vi "Otsu分割算法.vi"() -> ()   [LabVIEW 2018]
uses:
  <vilib>/Utility/error.llb/DialogType.ctl
  <vilib>/vision/NI_Vision_Development_Module.lvlib
  Dll/Otsu.dll
panel:
  in  "保存":bool
  out "像素当量单位":string
  out "像素当量":string
  out "是否进行像素标定":bool
  in  "单帧回看":bool
  out "火焰帧数":string
  in  "重新选择":bool
  in  "火焰详细参数":bool
  out "叠加部分":string
  out "单帧部分":string
  out "原图":T1(plugin-control)
  in  "返回主界面":bool
  in  "程序停止":bool
  out "Progress Bar":i32(slide) max=241 scale=-1.0..241.0
  out "单帧火焰":T1(plugin-control)
  out "叠加火焰":T1(plugin-control)
  # "基于Otsu算法的炮口火焰分割"
  # "火\n焰\n参\n数"
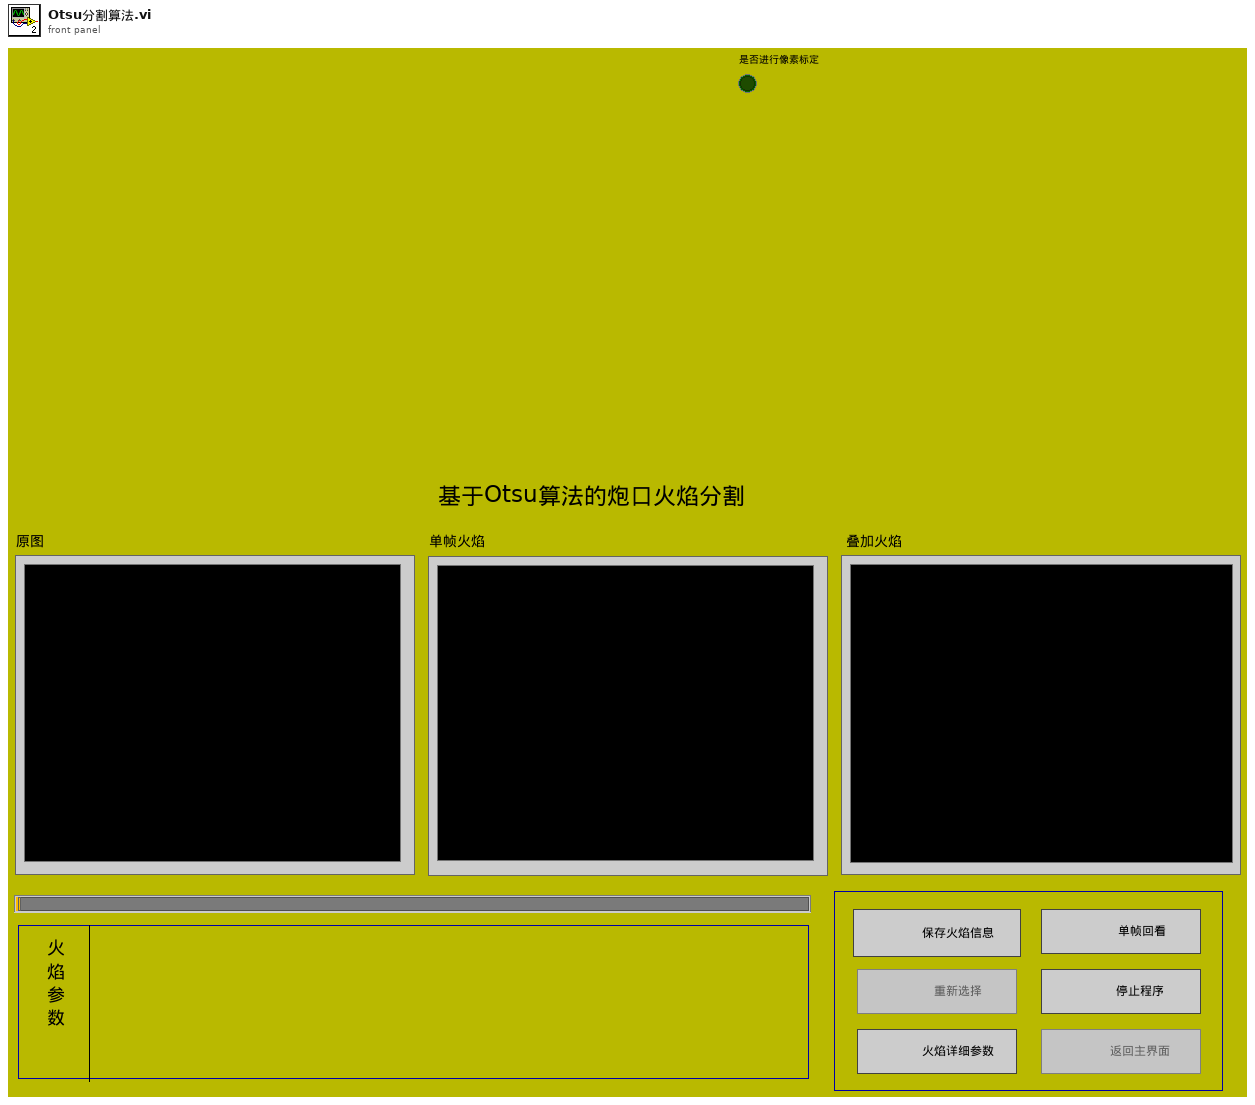
[diagram p1: front panel]
types:
  T1 = typedef "IMAQ Image.ctl" = refnum<image>
  T2 = enum8{"Enabled", "Disabled", "Disabled and Grayed Out"}
  T3 = enum32{"Invalid", "Standard", "Closed", "Hidden", "Minimized", "Maximized"}
  T4 = typedef "DialogType.ctl" = u16
  T5 = typedef "Image Type" = u32
  T6 = typedef "IMAQ AVI2 Refnum.ctl" = refnum<k20>
  T7 = cluster{"Width":u32, "Height":u32, "Frames Per Second":u32, "Codec":string, "Has Data":bool}
  T8 = typedef "ROI Descriptor" = cluster{"Global Rectangle":i32[], "Contours":cluster{"ID":enum32{"External", "Internal"}, "Type":u32, "Coordinates":i32[]}[]}
  T9 = cluster{"Area":dbl, "Number of Holes":dbl, "Bounding Rect":cluster{"Left":dbl, "Top":dbl, "Right":dbl, "Bottom":dbl}, "Center of Mass":cluster{"X":dbl, "Y":dbl}, "Orientation":dbl, "Dimensions":cluster{"Width":dbl, "Height":dbl}}[]
  T10 = cluster{"Particle Reports (Pixels)[0]":cluster{"Area":dbl, "Number of Holes":dbl, "Bounding Rect":cluster{"Left":dbl, "Top":dbl, "Right":dbl, "Bottom":dbl}, "Center of Mass":cluster{"X":dbl, "Y":dbl}, "Orientation":dbl, "Dimensions":cluster{"Width":dbl, "Height":dbl}}, "Particle Reports (Pixels)[1]":cluster{"Area":dbl, "Number of Holes":dbl, "Bounding Rect":cluster{"Left":dbl, "Top":dbl, "Right":dbl, "Bottom":dbl}, "Center of Mass":cluster{"X":dbl, "Y":dbl}, "Orientation":dbl, "Dimensions":cluster{"Width":dbl, "Height":dbl}}, "Particle Reports (Pixels)[2]":cluster{"Area":dbl, "Number of Holes":dbl, "Bounding Rect":cluster{"Left":dbl, "Top":dbl, "Right":dbl, "Bottom":dbl}, "Center of Mass":cluster{"X":dbl, "Y":dbl}, "Orientation":dbl, "Dimensions":cluster{"Width":dbl, "Height":dbl}}, "Particle Reports (Pixels)[3]":cluster{"Area":dbl, "Number of Holes":dbl, "Bounding Rect":cluster{"Left":dbl, "Top":dbl, "Right":dbl, "Bottom":dbl}, "Center of Mass":cluster{"X":dbl, "Y":dbl}, "Orientation":dbl, "Dimensions":cluster{"Width":dbl, "Height":dbl}}, "Particle Reports (Pixels)[4]":cluster{"Area":dbl, "Number of Holes":dbl, "Bounding Rect":cluster{"Left":dbl, "Top":dbl, "Right":dbl, "Bottom":dbl}, "Center of Mass":cluster{"X":dbl, "Y":dbl}, "Orientation":dbl, "Dimensions":cluster{"Width":dbl, "Height":dbl}}, "Particle Reports (Pixels)[5]":cluster{"Area":dbl, "Number of Holes":dbl, "Bounding Rect":cluster{"Left":dbl, "Top":dbl, "Right":dbl, "Bottom":dbl}, "Center of Mass":cluster{"X":dbl, "Y":dbl}, "Orientation":dbl, "Dimensions":cluster{"Width":dbl, "Height":dbl}}, "Particle Reports (Pixels)[6]":cluster{"Area":dbl, "Number of Holes":dbl, "Bounding Rect":cluster{"Left":dbl, "Top":dbl, "Right":dbl, "Bottom":dbl}, "Center of Mass":cluster{"X":dbl, "Y":dbl}, "Orientation":dbl, "Dimensions":cluster{"Width":dbl, "Height":dbl}}, "Particle Reports (Pixels)[7]":cluster{"Area":dbl, "Number of Holes":dbl, "Bounding Rect":cluster{"Left":dbl, "Top":dbl, "Right":dbl, "Bottom":dbl}, "Center of Mass":cluster{"X":dbl, "Y":dbl}, "Orientation":dbl, "Dimensions":cluster{"Width":dbl, "Height":dbl}}, "Particle Reports (Pixels)[8]":cluster{"Area":dbl, "Number of Holes":dbl, "Bounding Rect":cluster{"Left":dbl, "Top":dbl, "Right":dbl, "Bottom":dbl}, "Center of Mass":cluster{"X":dbl, "Y":dbl}, "Orientation":dbl, "Dimensions":cluster{"Width":dbl, "Height":dbl}}}
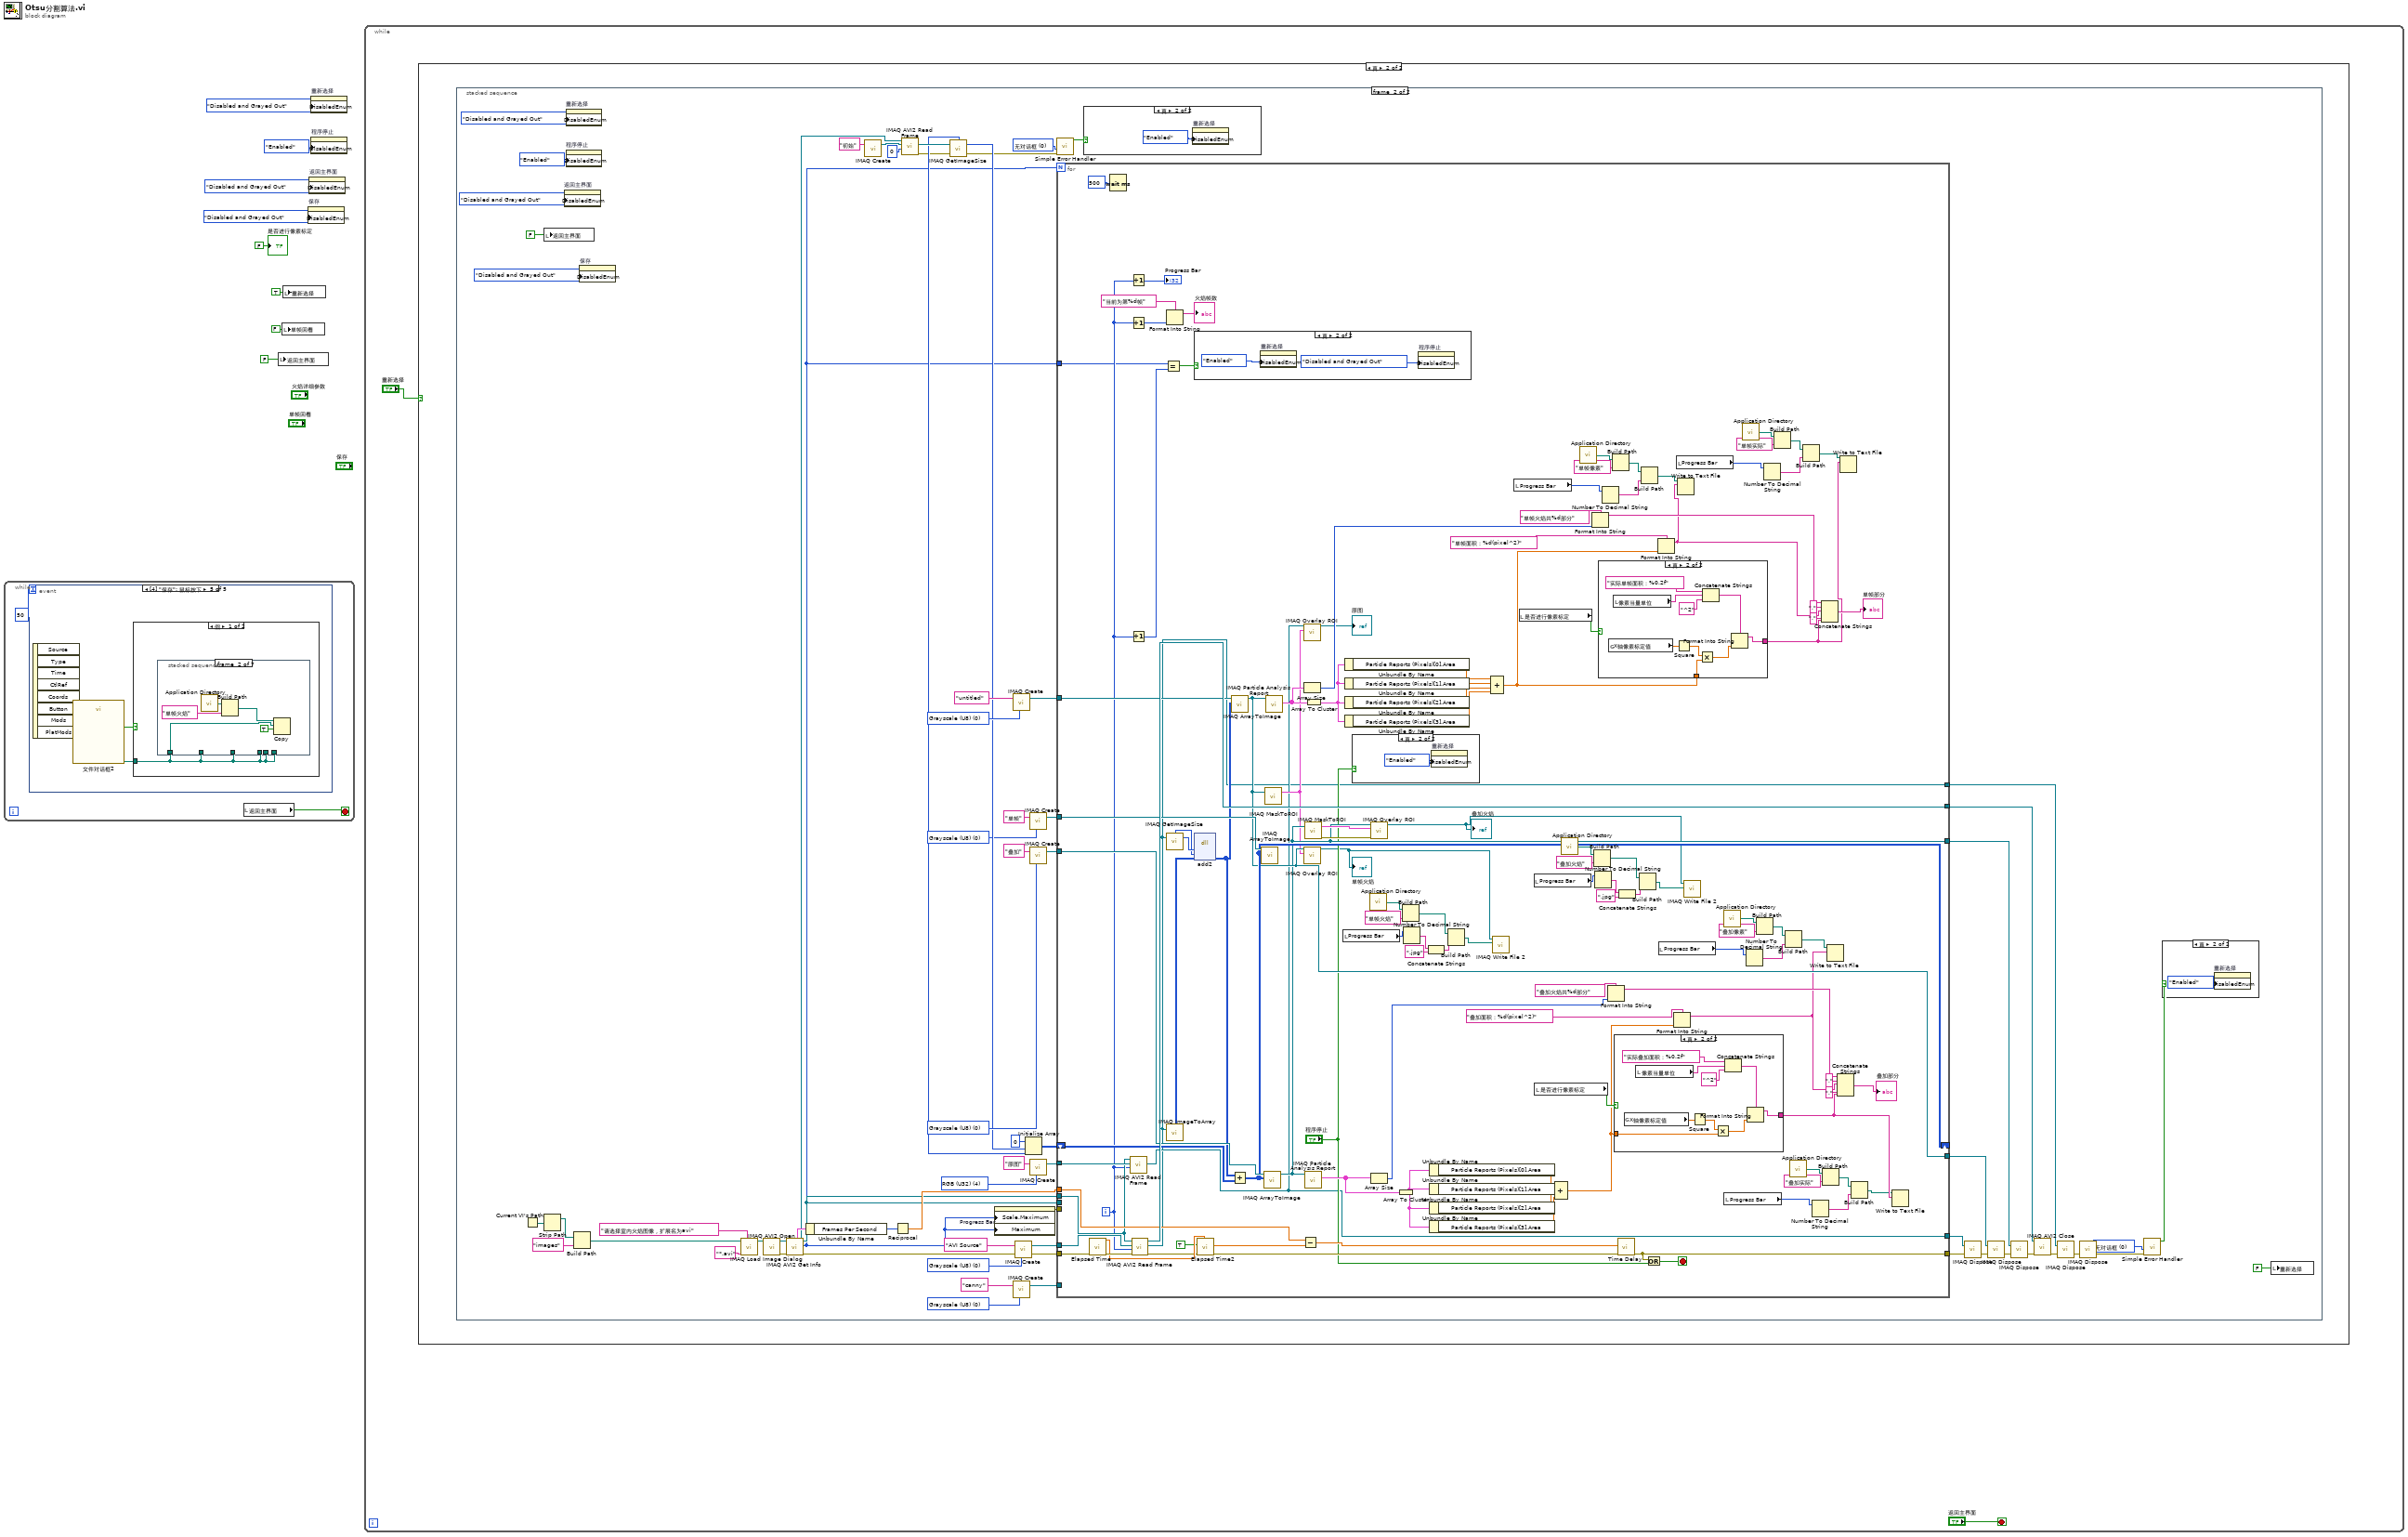
[diagram p0: block diagram]
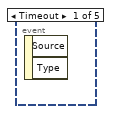
[diagram p2: hidden frame]
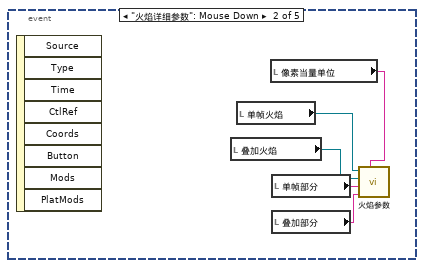
[diagram p3: hidden frame]
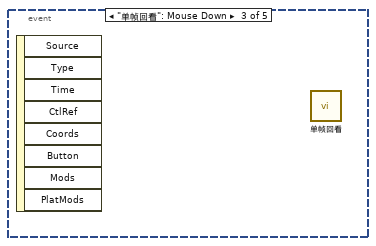
[diagram p4: hidden frame]
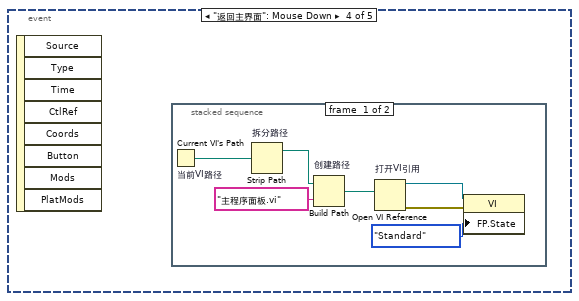
[diagram p5: hidden frame]
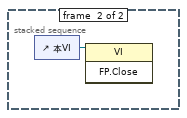
[diagram p6: hidden frame]
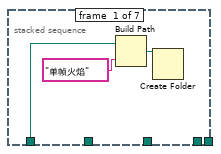
[diagram p7: hidden frame]
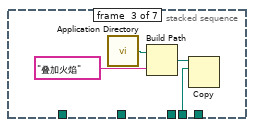
[diagram p8: hidden frame]
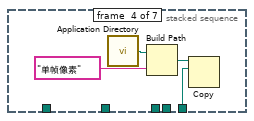
[diagram p9: hidden frame]
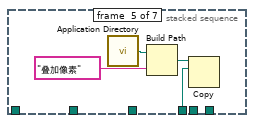
[diagram p10: hidden frame]
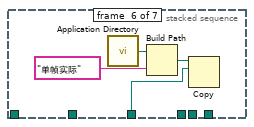
[diagram p11: hidden frame]
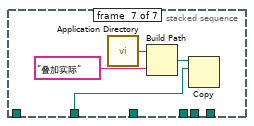
[diagram p12: hidden frame]
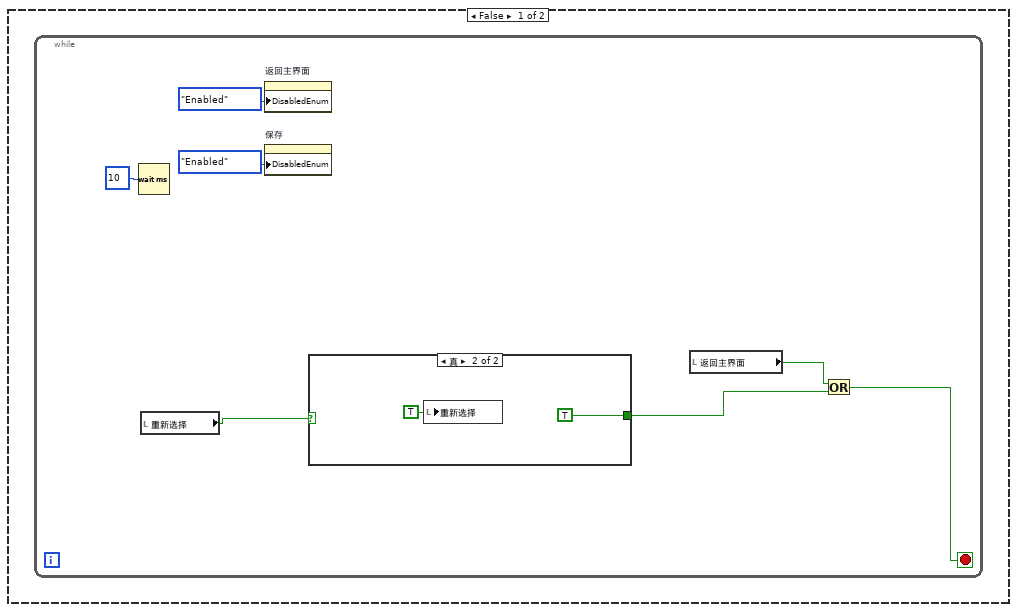
[diagram p14: hidden frame]
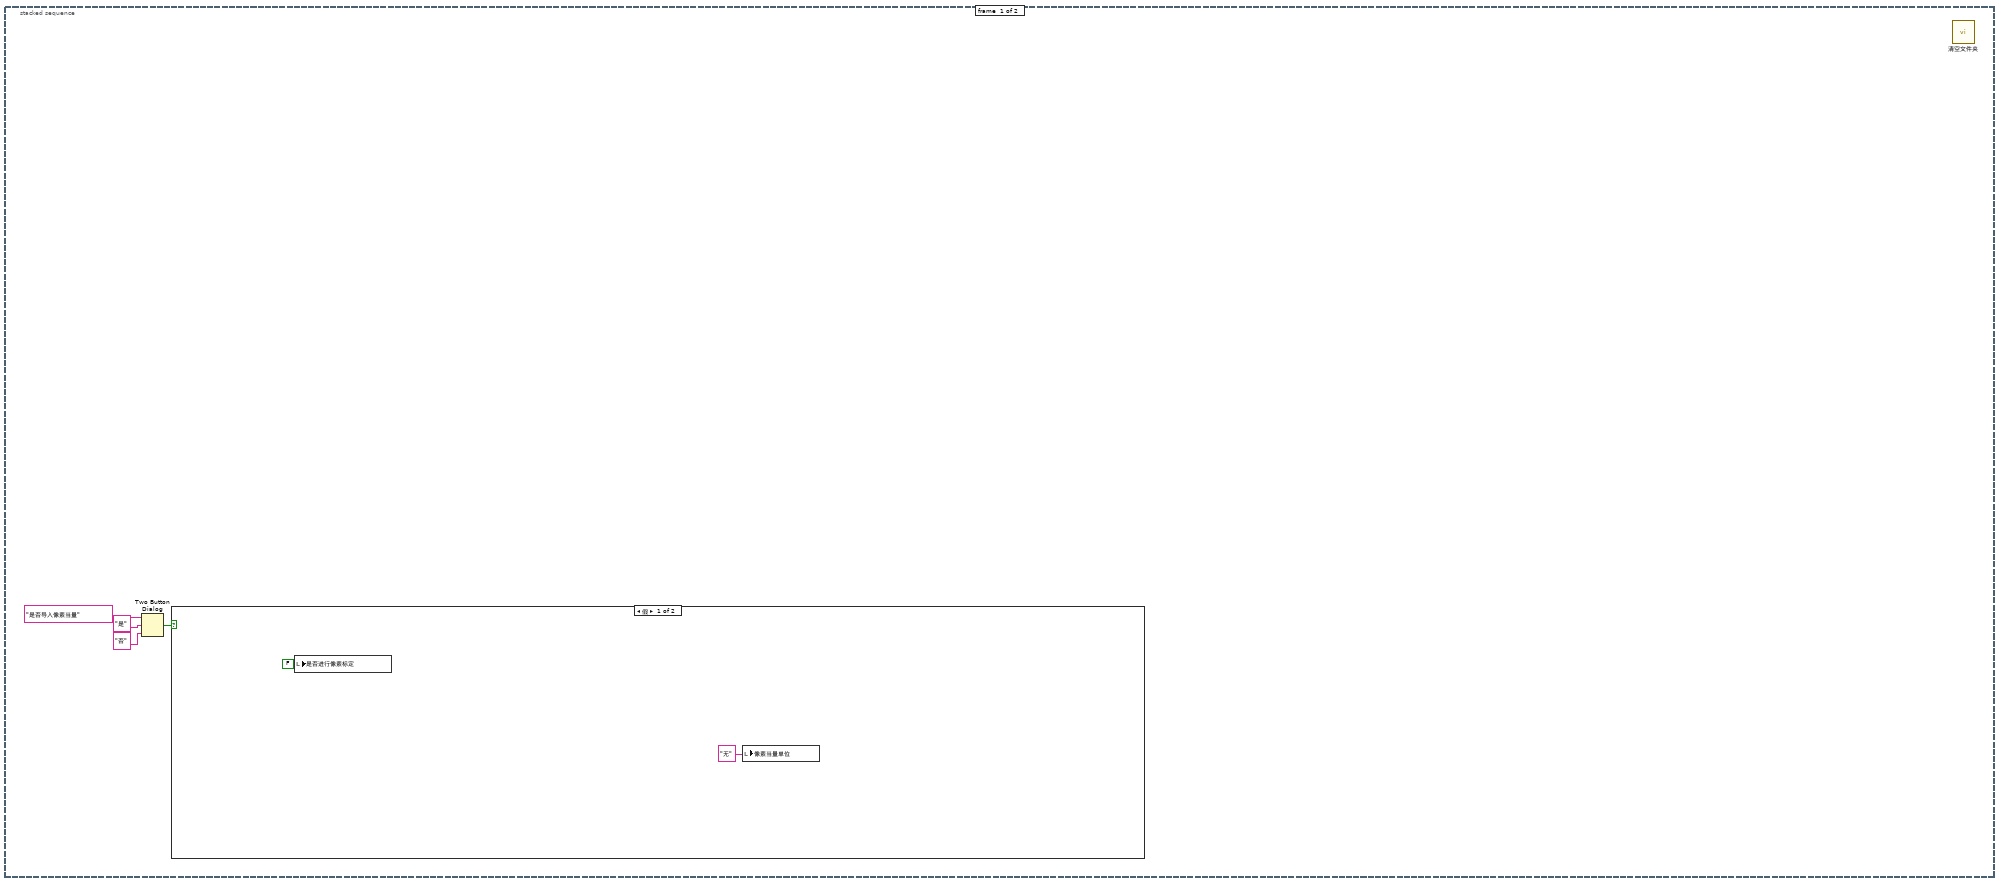
[diagram p16: hidden frame]
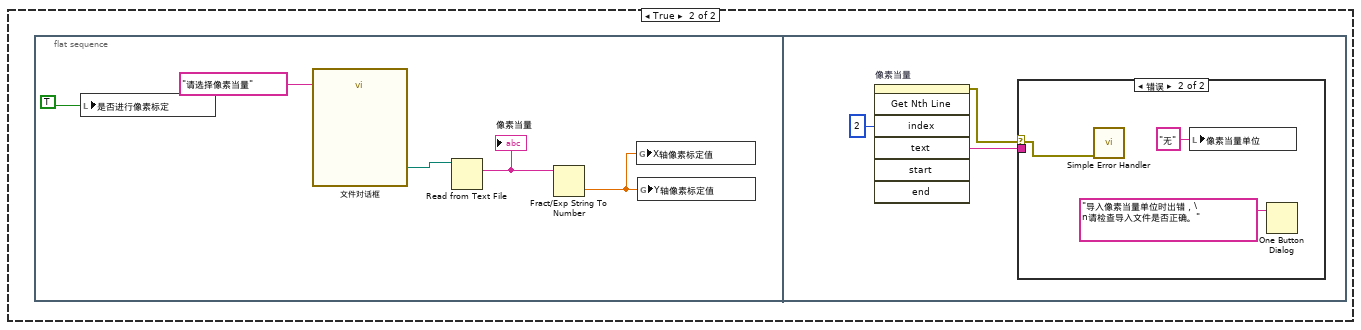
[diagram p17: hidden frame]
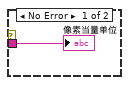
[diagram p18: hidden frame]
diagram:
  n1 = while {
    stop <- w10 stop-if-true
    n2 = event shown="[4] \"保存\": 鼠标按下" {
      selector: _ -> [_ _ _ _ _]
      dyn-events: _ -> [_ _ _ _ _]
      timeout: 50 -> [_ _ _ _ _]
      event Timeout {
        n3 = event-data() -> ()  [unwired: 1 in, 2 out]
      }
      event "火焰详细参数": Mouse Down {
        n4 = event-data() -> ()  [unwired: 1 in, 8 out]
        n5 = local read "叠加火焰"() -> (w12:T1)
        n6 = local read "单帧火焰"() -> (w13:T1)
        n7 = local read "像素当量单位"() -> (w11:string)
        n8 = local read "单帧部分"() -> (w15:string)
        n9 = local read "叠加部分"() -> (w14:string)
        n10 = call "火焰参数.vi"("像素当量单位"=w11, 8:w14, 9:w15, "Image 2"=w12, "Image"=w13) -> ()  [unwired: 7 in]
      }
      event "单帧回看": Mouse Down {
        n11 = event-data() -> ()  [unwired: 1 in, 8 out]
        n12 = call "单帧回看.vi"() -> ()  [unwired: 28 in]
      }
      event "返回主界面": Mouse Down {
        n13 = event-data() -> ()  [unwired: 1 in, 8 out]
        n14 = stacked-sequence {
          frame #0 {
            n15 = Current VI's Path "当前VI路径"() -> (path=w20:path)
            n16 = Strip Path "拆分路径"(path=w20) -> (stripped path=w22:path)  [unwired: 1 out]
            n17 = Build Path "创建路径"(base path=w22, name or relative path="主程序面板.vi" ("名称或相对路径")) -> (appended path=w21:path)
            n18 = Open VI Reference "打开VI引用"(vi path=w21) -> (vi reference=w19:refnum<vi>, error out=w18:errorcluster)  [unwired: 5 in]
            n19 = property class="VI"(reference=w19, error in=w18, "FP.State"=T3."Standard" ("前面板窗口:状态")) -> ()  [unwired: 2 out]
          }
          frame #1 {
            n20 = control-ref of="本VI"() -> (w23:refnum<vi>)
            n21 = invoke class="VI" method="FP.Close"(reference=w23) -> ()  [unwired: 2 in, 3 out]
          }
        }
      }
      event "保存": Mouse Down {
        n22 = event-data() -> ()  [unwired: 1 in, 8 out]
        n23 = call "文件对话框2"() -> ("selected path"=w24:path, "cancelled"=w25:bool)  [unwired: 12 in, 2 out]
        n24 = case shown="假" w25 {
          tunnel: w24 -> [w26 _]
          frame False {
            n25 = stacked-sequence {
              tunnel: w26 -> [w27 w31 _ _ _ _ _]
              tunnel: w26 -> [_ _ w36 _ _ _ _]
              tunnel: w26 -> [_ _ _ w40 _ _ _]
              tunnel: w26 -> [_ _ _ _ w44 _ _]
              tunnel: w26 -> [_ _ _ _ _ w48 _]
              tunnel: w26 -> [_ _ _ _ _ _ w51]
              frame #0 {
                n26 = Build Path(base path=w27, name or relative path="单帧火焰" ("名称或相对路径")) -> (appended path=w29:path)
                n27 = Create Folder(path (use dialog)=w29) -> ()  [unwired: 2 in, 3 out]
              }
              frame #1 {
                n28 = call <vilib>:"Application Directory.vi"() -> ("Application Directory"=w34:path)
                n29 = Build Path(base path=w34, name or relative path="单帧火焰" ("名称或相对路径")) -> (appended path=w32:path)
                n30 = Copy(9:TRUE ("覆盖(F)"), 10:w31, 11:w32) -> ()  [unwired: 2 in, 3 out]
              }
              frame #2 {
                n31 = call <vilib>:"Application Directory.vi"() -> ("Application Directory"=w37:path)
                n32 = Build Path(base path=w37, name or relative path="叠加火焰" ("名称或相对路径")) -> (appended path=w38:path)
                n33 = Copy(10:w36, 11:w38) -> ()  [unwired: 3 in, 3 out]
              }
              frame #3 {
                n34 = call <vilib>:"Application Directory.vi"() -> ("Application Directory"=w41:path)
                n35 = Build Path(base path=w41, name or relative path="单帧像素" ("名称或相对路径")) -> (appended path=w42:path)
                n36 = Copy(10:w40, 11:w42) -> ()  [unwired: 3 in, 3 out]
              }
              frame #4 {
                n37 = call <vilib>:"Application Directory.vi"() -> ("Application Directory"=w45:path)
                n38 = Build Path(base path=w45, name or relative path="叠加像素" ("名称或相对路径")) -> (appended path=w46:path)
                n39 = Copy(10:w44, 11:w46) -> ()  [unwired: 3 in, 3 out]
              }
              frame #5 {
                n40 = call <vilib>:"Application Directory.vi"() -> ("Application Directory"=w49:path)
                n41 = Build Path(base path=w49, name or relative path="单帧实际" ("名称或相对路径")) -> (appended path=w50:path)
                n42 = Copy(10:w48, 11:w50) -> ()  [unwired: 3 in, 3 out]
              }
              frame #6 {
                n43 = call <vilib>:"Application Directory.vi"() -> ("Application Directory"=w53:path)
                n44 = Build Path(base path=w53, name or relative path="叠加实际" ("名称或相对路径")) -> (appended path=w54:path)
                n45 = Copy(10:w51, 11:w54) -> ()  [unwired: 3 in, 3 out]
              }
            }
          }
          frame True {
          }
        }
      }
    }
    n46 = local read "返回主界面"() -> (w10:bool)
  }
  n47 = local write "返回主界面"(FALSE ("重新选择")) -> ()
  n48 = local write "单帧回看"(FALSE ("重新选择")) -> ()
  n49 = local write "重新选择"(TRUE ("重新选择")) -> ()
  n50 = property on="保存" class="Bool (严格)"("DisabledEnum"=T2."Disabled and Grayed Out" ("禁用")) -> ()  [unwired: 2 in, 2 out]
  n51 = property on="返回主界面" class="Bool (严格)"("DisabledEnum"=T2."Disabled and Grayed Out" ("禁用")) -> ()  [unwired: 2 in, 2 out]
  n52 = property on="重新选择" class="Bool (严格)"("DisabledEnum"=T2."Disabled and Grayed Out" ("禁用")) -> ()  [unwired: 2 in, 2 out]
  n53 = property on="程序停止" class="Bool"("DisabledEnum"=T2."Enabled" ("禁用")) -> ()  [unwired: 2 in, 2 out]
  n54 = while {
    stop <- "返回主界面" stop-if-true
    n55 = case shown="真" "重新选择" {
      frame False {
        n56 = while {
          stop <- w59 stop-if-true
          n57 = Wait (ms)(milliseconds to wait=u32 10 ("等待时间（毫秒）")) -> ()  [unwired: 1 out]
          n58 = local read "重新选择"() -> (w62:bool)
          n59 = property on="返回主界面" class="Bool (严格)"("DisabledEnum"=T2."Enabled" ("禁用")) -> ()  [unwired: 2 in, 2 out]
          n60 = property on="保存" class="Bool (严格)"("DisabledEnum"=T2."Enabled" ("禁用")) -> ()  [unwired: 2 in, 2 out]
          n61 = case shown="真" w62 {
            tunnel: [_ TRUE] -> w60
            frame False {
            }
            frame True {
              n62 = local write "重新选择"(TRUE ("重新选择")) -> ()
            }
          }
          n63 = local read "返回主界面"() -> (w61:bool)
          n64 = Or(x=w61, y=w60) -> (x .or. y?=w59:bool)
        }
      }
      frame True {
        n65 = stacked-sequence {
          frame #0 {
            n66 = Two Button Dialog(message="是否导入像素当量" ("消息"), 1:"否" ("F按钮名称（“取消”）"), 2:"是" ("T按钮名称（“确定”）")) -> (T button?=w69:bool)
            n67 = case shown="假" w69 {
              frame False {
                n68 = local write "是否进行像素标定"(FALSE ("是否进行像素标定")) -> ()
                n69 = local write "像素当量单位"("无" ("像素当量单位")) -> ()
              }
              frame True {
                n70 = flat-sequence {
                  frame #0 {
                    n71 = local write "是否进行像素标定"(TRUE ("是否进行像素标定")) -> ()
                    n72 = call "文件对话框"("default name"="请选择像素当量") -> ("selected path"=w74:path)  [unwired: 11 in, 3 out]
                    n73 = Read from Text File(file (use dialog)=w74) -> (text=w75:string)  [unwired: 3 in, 3 out]
                    "像素当量" <- w75
                    n74 = Fract/Exp String To Number(string=w75) -> (number=w76:dbl)  [unwired: 3 in, 1 out]
                    n75 = global write "全局变量.vi" "X轴像素标定值"(w76) -> ()
                    n76 = global write "全局变量.vi" "Y轴像素标定值"(w76) -> ()
                  }
                  frame #1 {
                    n77 = invoke on="像素当量" class="Str" method="Get Nth Line"("index"=u32 2 ("行索引")) -> (error out=w77:errorcluster, "text"=w78:string)  [unwired: 6 in, 5 out]
                    n78 = case shown="错误" w77 {
                      selector: w77 -> [_ w83]
                      tunnel: w78 -> [w80 _]
                      frame No Error {
                        "像素当量单位" <- w80
                      }
                      frame Error {
                        n79 = call <vilib>:"Simple Error Handler.vi"("error in (no error)"=w83) -> ()  [unwired: 4 in, 5 out]
                        n80 = local write "像素当量单位"("无" ("像素当量单位")) -> ()
                        n81 = One Button Dialog(message="导入像素当量单位时出错，\n请检查导入文件是否正确。" ("消息")) -> ()  [unwired: 1 in, 1 out]
                      }
                    }
                  }
                }
              }
            }
            n82 = call "清空文件夹.vi"() -> ()  [unwired: 12 in]
          }
          frame #1 {
            w94 = T4 0 items=["无对话框", "确定信息", "继续或停止信息", "确定信息＋警告", "继续/停止+警告"] ("type of dialog (OK msg:1)")
            w95 = T4 0 items=["无对话框", "确定信息", "继续或停止信息", "确定信息＋警告", "继续/停止+警告"] ("type of dialog (OK msg:1)")
            w106 = T5 0 items=["Grayscale (U8)", "Grayscale (I16)", "Grayscale (SGL)", "Complex (CSG)", "RGB (U32)", "HSL (U32)", "RGB (U64)", "Grayscale (U16)"] ("Image Type")
            w107 = T5 4 items=["Grayscale (U8)", "Grayscale (I16)", "Grayscale (SGL)", "Complex (CSG)", "RGB (U32)", "HSL (U32)", "RGB (U64)", "Grayscale (U16)"] ("Image Type")
            w111 = T5 0 items=["Grayscale (U8)", "Grayscale (I16)", "Grayscale (SGL)", "Complex (CSG)", "RGB (U32)", "HSL (U32)", "RGB (U64)", "Grayscale (U16)"] ("Image Type")
            w132 = T5 0 items=["Grayscale (U8)", "Grayscale (I16)", "Grayscale (SGL)", "Complex (CSG)", "RGB (U32)", "HSL (U32)", "RGB (U64)", "Grayscale (U16)"] ("Image Type")
            w136 = T5 0 items=["Grayscale (U8)", "Grayscale (I16)", "Grayscale (SGL)", "Complex (CSG)", "RGB (U32)", "HSL (U32)", "RGB (U64)", "Grayscale (U16)"] ("Image Type")
            w137 = T5 0 items=["Grayscale (U8)", "Grayscale (I16)", "Grayscale (SGL)", "Complex (CSG)", "RGB (U32)", "HSL (U32)", "RGB (U64)", "Grayscale (U16)"] ("Image Type")
            n83 = Current VI's Path() -> (path=w90:path)
            n84 = local write "返回主界面"(FALSE ("重新选择")) -> ()
            n85 = Strip Path(path=w90) -> (stripped path=w91:path)  [unwired: 1 out]
            n86 = property on="返回主界面" class="Bool (严格)"("DisabledEnum"=T2."Disabled and Grayed Out" ("禁用")) -> ()  [unwired: 2 in, 2 out]
            n87 = property on="重新选择" class="Bool (严格)"("DisabledEnum"=T2."Disabled and Grayed Out" ("禁用")) -> ()  [unwired: 2 in, 2 out]
            n88 = property on="程序停止" class="Bool"("DisabledEnum"=T2."Enabled" ("禁用")) -> ()  [unwired: 2 in, 2 out]
            n89 = Build Path(base path=w91, name or relative path="images") -> (appended path=w88:path)
            n90 = property on="保存" class="Bool (严格)"("DisabledEnum"=T2."Disabled and Grayed Out" ("禁用")) -> ()  [unwired: 2 in, 2 out]
            n91 = call "IMAQ Load Image Dialog"("Prompt"="请选择室内火焰图像，扩展名为avi" ("prompt"), "Pattern"="*.avi", "Start Path"=w88) -> ("Path"=w119:path)  [unwired: 6 in, 2 out]
            n92 = call "IMAQ AVI2 Open"("AVI File Path"=w119) -> ("error out"=w148:errorcluster, "AVI Refnum"=w147:T6)  [unwired: 2 in, 7 out]
            n93 = call "IMAQ AVI2 Get Info"("error in (no error)"=w148, "AVI Refnum"=w147) -> ("error out"=w145:errorcluster, "Number of Frames"=w98:u32, "AVI Refnum (duplicate)"=w123:T6, "Frame Data"=w149:T7)  [unwired: 6 out]
            n94 = Unbundle By Name(w149) -> ("Frames Per Second"=w140:u32)
            n95 = call "IMAQ Create"("Image Name"="初始") -> ("New Image"=w129:T1)  [unwired: 4 in, 1 out]
            n96 = Reciprocal(x=w140) -> (1/x=w139:dbl)
            n97 = call "IMAQ AVI2 Read Frame"("Frame Number"=u32 0, "Image"=w129, "AVI Refnum"=w123) -> ("error out"=w97:errorcluster, "Image Out"=w127:T1)  [unwired: 1 in, 6 out]
            n98 = call "IMAQ GetImageSize"("Image"=w127, "error in (no error)"=w97) -> ("Y Resolution"=w126:i32, "X Resolution"=w122:i32, "error out"=w96:errorcluster)  [unwired: 2 in]
            n99 = property on="Progress Bar" class="Slide (严格)"("Scale.Maximum"=w98, "Maximum"=w98) -> (error out=w138:errorcluster)  [unwired: 2 in, 1 out]
            n100 = call "IMAQ Create"("Image Name"="untitled", "Image Type"=w136) -> ("New Image"=w135:T1)  [unwired: 2 in, 2 out]
            n101 = call "IMAQ Create"("Image Name"="canny", "Image Type"=w106) -> ("New Image"=w104:T1)  [unwired: 2 in, 2 out]
            n102 = call "IMAQ Create"("Image Name"="AVI Source", "Image Type"=w137, "error in (no error)"=w145) -> ("New Image"=w143:T1, "error out"=w144:errorcluster)  [unwired: 1 in, 1 out]
            n103 = Initialize Array(u8 0 ("元素"), w126, w122) -> (w124:u8[][])
            n104 = call "IMAQ Create"("Image Name"="单帧", "Image Type"=w111) -> ("New Image"=w113:T1)  [unwired: 3 in, 1 out]
            n105 = call "IMAQ Create"("Image Name"="叠加", "Image Type"=w132) -> ("New Image"=w131:T1)  [unwired: 3 in, 1 out]
            n106 = call "IMAQ Create"("Image Name"="原图", "Image Type"=w107) -> ("New Image"=w109:T1)  [unwired: 2 in, 2 out]
            n107 = call <vilib>:"Simple Error Handler.vi"("type of dialog (OK msg:1)"=w95, "error in (no error)"=w96) -> ("error?"=w92:bool)  [unwired: 3 in, 4 out]
            n108 = for {
              N: w98 -> [_]
              tunnel: w143 -> [w270]
              tunnel: [w269] -> w146
              tunnel: [w260] -> w103
              tunnel: w144 -> [w268]
              tunnel: w123 -> [w246]
              tunnel: [w218] -> w141
              tunnel: w139 -> [w266]
              tunnel: w138 -> [_]
              tunnel: w135 -> [w250]
              tunnel: w131 -> [w256]
              shift-right: [w249] -> _
              shift-left: w124 -> [w255]
              tunnel: w123 -> [_]
              tunnel: [w231] -> w118
              tunnel: w113 -> [w251]
              tunnel: [w234] -> w110
              tunnel: w109 -> [w247]
              tunnel: w104 -> [_]
              tunnel: [w219] -> w101
              tunnel: w98 -> [w221]
              i -> [w222]
              stop <- w259 stop-if-true
              n109 = call "Elapsed Time"("error in (no error)"=w268) -> ("Present (s)"=w264:dbl, "error out"=w267:errorcluster)  [unwired: 11 in, 6 out]
              n110 = Wait (ms)(milliseconds to wait=u32 500) -> ()  [unwired: 1 out]
              n111 = call "IMAQ AVI2 Read Frame"("Frame Number"=w222, "Image"=w247, "AVI Refnum"=w246) -> ("Image Out"=w219:T1)  [unwired: 1 in, 7 out]
              n112 = Increment(x=w222) -> (x+1=→"Progress Bar":i32)
              n113 = Increment(x=w222) -> (x+1=w226:i32)
              n114 = Increment(x=w222) -> (x+1=w220:i32)
              n115 = call "IMAQ AVI2 Read Frame"("error in (no error)"=w267, "Frame Number"=w222, "Image"=w270, "AVI Refnum"=w246) -> ("error out"=w262:errorcluster, "Image Out"=w218:T1, "AVI Refnum (duplicate)"=w269:T6)  [unwired: 5 out]
              n116 = Equal?(x=w221, y=w220) -> (x = y?=w223:bool)
              n117 = Format Into String(format string="当前为第%d帧" ("格式字符串"), w226) -> (resulting string=→"火焰帧数":string)  [unwired: 2 in, 1 out]
              n118 = call "IMAQ GetImageSize"("Image"=w218) -> ("Y Resolution"=w254:i32, "X Resolution"=w253:i32)  [unwired: 3 in, 1 out]
              n119 = call "IMAQ ImageToArray"("Image"=w218) -> ("Image Pixels (U8)"=w252:u8[][])  [unwired: 3 in, 4 out]
              n120 = case shown="真" w223 {
                frame False {
                }
                frame True {
                  n121 = property on="重新选择" class="Bool (严格)"("DisabledEnum"=T2."Enabled" ("禁用")) -> ()  [unwired: 2 in, 2 out]
                  n122 = property on="程序停止" class="Bool"("DisabledEnum"=T2."Disabled and Grayed Out" ("禁用")) -> ()  [unwired: 2 in, 2 out]
                }
              }
              n123 = dll-call lib="PTH2<abs DsdhProgramme_GuShiJu火焰分割DllOtsu.dll" fn="add2"("rows"=w254, "cols"=w253, "data"=w252) -> ("data"=w248:u8[][])  [unwired: 6 in, 2 out]
              n124 = call "Elapsed Time2"("Reset"=TRUE, "error in (no error)"=w262, "Set Start Time (s)"=w264) -> ("Elapsed Time (s)"=w261:dbl, "error out"=w228:errorcluster)  [unwired: 9 in, 6 out]
              n125 = call "IMAQ ArrayToImage"("Image Pixels (U8)"=w248, "Image"=w250) -> ("Image Out"=w234:T1)  [unwired: 8 in, 1 out]
              n126 = Add(x=w248, y=w255) -> (x+y=w249:u8[][])
              n127 = call "IMAQ ArrayToImage"("Image Pixels (U8)"=w249, "Image"=w251) -> ()  [unwired: 8 in, 2 out]
              n128 = call "IMAQ ArrayToImage"("Image Pixels (U8)"=w249, "Image"=w256) -> ("Image Out"=w231:T1)  [unwired: 8 in, 1 out]
              n129 = call "IMAQ MaskToROI"("Image"=w234) -> ("ROI Descriptor"=w229:T8)  [unwired: 6 in, 2 out]
              n130 = call "IMAQ Particle Analysis Report"("Image"=w234) -> ("Particle Reports (Pixels)"=w236:T9)  [unwired: 5 in, 5 out]
              n131 = Subtract(x=w266, y=w261) -> (x-y=w265:dbl)
              n132 = call "IMAQ Overlay ROI"("ROI Descriptor"=w229, "Image"=w219) -> ("Image Out"=→"原图":T1)  [unwired: 8 in, 1 out]
              n133 = Array Size(array=w236) -> (size(s)=w237:i32)
              n134 = call "IMAQ Overlay ROI"("ROI Descriptor"=w229, "Image"=w234) -> ("Image Out"=w209:T1)  [unwired: 8 in, 1 out]
              "单帧火焰" <- w209
              n135 = call "IMAQ MaskToROI"("Image"=w231) -> ("ROI Descriptor"=w232:T8, "error out"=w233:errorcluster)  [unwired: 6 in, 1 out]
              n136 = call "IMAQ Particle Analysis Report"("Image"=w231) -> ("Particle Reports (Pixels)"=w235:T9)  [unwired: 5 in, 5 out]
              n137 = Array To Cluster(array=w236) -> (cluster=w216:T10)
              n138 = local read "Progress Bar"() -> (w208:i32)
              n139 = Unbundle By Name(w216) -> ("Particle Reports (Pixels)[0].Area"=w245:dbl)
              n140 = Unbundle By Name(w216) -> ("Particle Reports (Pixels)[1].Area"=w244:dbl)
              n141 = Unbundle By Name(w216) -> ("Particle Reports (Pixels)[2].Area"=w243:dbl)
              n142 = Unbundle By Name(w216) -> ("Particle Reports (Pixels)[3].Area"=w242:dbl)
              n143 = case shown="真" "程序停止" {
                frame False {
                }
                frame True {
                  n144 = property on="重新选择" class="Bool (严格)"("DisabledEnum"=T2."Enabled" ("禁用")) -> ()  [unwired: 2 in, 2 out]
                }
              }
              n145 = call <vilib>:"Application Directory.vi"() -> ("Application Directory"=w214:path)
              n146 = call "IMAQ Overlay ROI"("error in (no error)"=w233, "ROI Descriptor"=w232, "Image"=w231) -> ("Image Out"=w197:T1)  [unwired: 7 in, 1 out]
              "叠加火焰" <- w197
              n147 = Array Size(array=w235) -> (size(s)=w184:i32)
              n148 = Array To Cluster(array=w235) -> (cluster=w217:T10)
              n149 = Build Path(base path=w214, name or relative path="单帧火焰" ("名称或相对路径")) -> (appended path=w212:path)
              n150 = Number To Decimal String(number=w208) -> (decimal integer string=w207:string)  [unwired: 1 in]
              n151 = Concatenate Strings(w207, ".jpg" ("字符串")) -> (w211:string)
              n152 = Unbundle By Name(w217) -> ("Particle Reports (Pixels)[0].Area"=w241:dbl)
              n153 = Unbundle By Name(w217) -> ("Particle Reports (Pixels)[1].Area"=w240:dbl)
              n154 = Unbundle By Name(w217) -> ("Particle Reports (Pixels)[2].Area"=w239:dbl)
              n155 = Unbundle By Name(w217) -> ("Particle Reports (Pixels)[3].Area"=w215:dbl)
              n156 = Build Path(base path=w212, name or relative path=w211) -> (appended path=w206:path)
              n157 = Compound Arithmetic op=ADD(w245, w244, w243, w242) -> (w191:dbl)
              n158 = call-poly "IMAQ Write File 2"("File Path"=w206, "Image"=w209) -> ()  [unwired: 8 in, 2 out]
              n159 = local read "Progress Bar"() -> (w179:i32)
              n160 = local read "是否进行像素标定"() -> (w194:bool)
              n161 = local read "Progress Bar"() -> (w203:i32)
              n162 = local read "是否进行像素标定"() -> (w188:bool)
              n163 = Compound Arithmetic op=ADD(w241, w240, w239, w215) -> (w183:dbl)
              n164 = call <vilib>:"Application Directory.vi"() -> ("Application Directory"=w198:path)
              n165 = call <vilib>:"Application Directory.vi"() -> ("Application Directory"=w182:path)
              n166 = Format Into String(format string="单帧火焰共%d部分" ("初始字符串"), w237) -> (resulting string=w195:string)  [unwired: 2 in, 1 out]
              n167 = Build Path(base path=w198, name or relative path="叠加火焰" ("名称或相对路径")) -> (appended path=w200:path)
              n168 = Number To Decimal String(number=w203) -> (decimal integer string=w204:string)  [unwired: 1 in]
              n169 = case shown="真" w194 {
                tunnel: ["未进行像素标定" ("初始字符串") w286] -> w170
                tunnel: w191 -> [_ w288]
                frame False {
                }
                frame True {
                  n170 = global read "全局变量.vi" "X轴像素标定值"() -> (w290:dbl)
                  n171 = local read "像素当量单位"() -> (w283:string)
                  n172 = Square(x=w290) -> (x^2=w289:dbl)
                  n173 = Multiply(x=w289, y=w288) -> (x*y=w287:dbl)
                  n174 = Concatenate Strings("实际单帧面积：%0.2f" ("初始字符串"), w283, "^2" ("字符串")) -> (w284:string)
                  n175 = Format Into String(format string=w284, w287) -> (resulting string=w286:string)  [unwired: 2 in, 1 out]
                }
              }
              n176 = Number To Decimal String(number=w179) -> (decimal integer string=w178:string)  [unwired: 1 in]
              n177 = Format Into String(format string="叠加火焰共%d部分" ("初始字符串"), w184) -> (resulting string=w187:string)  [unwired: 2 in, 1 out]
              n178 = Build Path(base path=w182, name or relative path="单帧像素" ("名称或相对路径")) -> (appended path=w180:path)
              n179 = case shown="真" w188 {
                tunnel: ["未进行像素标定" ("初始字符串") w277] -> w156
                tunnel: w183 -> [_ w276]
                frame False {
                }
                frame True {
                  n180 = global read "全局变量.vi" "X轴像素标定值"() -> (w280:dbl)
                  n181 = local read "像素当量单位"() -> (w274:string)
                  n182 = Square(x=w280) -> (x^2=w279:dbl)
                  n183 = Multiply(x=w279, y=w276) -> (x*y=w278:dbl)
                  n184 = Concatenate Strings("实际叠加面积：%0.2f" ("初始字符串"), w274, "^2" ("字符串")) -> (w272:string)
                  n185 = Format Into String(format string=w272, w278) -> (resulting string=w277:string)  [unwired: 2 in, 1 out]
                }
              }
              n186 = call "Time Delay"("error in (no error)"=w228, "Delay Time (s)"=w265) -> ("error out"=w260:errorcluster)  [unwired: 9 in]
              n187 = Concatenate Strings(w204, ".jpg" ("字符串")) -> (w201:string)
              n188 = Build Path(base path=w200, name or relative path=w201) -> (appended path=w205:path)
              n189 = Build Path(base path=w180, name or relative path=w178) -> (appended path=w176:path)
              n190 = Or(x=w260, y="程序停止") -> (x .or. y?=w259:bool)
              n191 = Format Into String(format string="单帧面积：%d(pixel^2)" ("初始字符串"), w191) -> (resulting string=w177:string)  [unwired: 2 in, 1 out]
              n192 = local read "Progress Bar"() -> (w163:i32)
              n193 = Format Into String(format string="叠加面积：%d(pixel^2)" ("初始字符串"), w183) -> (resulting string=w157:string)  [unwired: 2 in, 1 out]
              n194 = local read "Progress Bar"() -> (w174:i32)
              n195 = Write to Text File(file (use dialog)=w176, text=w177) -> ()  [unwired: 2 in, 3 out]
              n196 = call-poly "IMAQ Write File 2"("File Path"=w205, "Image"=w197) -> ()  [unwired: 8 in, 2 out]
              n197 = call <vilib>:"Application Directory.vi"() -> ("Application Directory"=w160:path)
              n198 = local read "Progress Bar"() -> (w164:i32)
              n199 = call <vilib>:"Application Directory.vi"() -> ("Application Directory"=w171:path)
              n200 = Number To Decimal String(number=w163) -> (decimal integer string=w159:string)  [unwired: 1 in]
              n201 = Build Path(base path=w160, name or relative path="叠加像素" ("名称或相对路径")) -> (appended path=w162:path)
              n202 = Number To Decimal String(number=w174) -> (decimal integer string=w169:string)  [unwired: 1 in]
              n203 = Build Path(base path=w171, name or relative path="单帧实际" ("名称或相对路径")) -> (appended path=w173:path)
              n204 = Build Path(base path=w162, name or relative path=w159) -> (appended path=w158:path)
              n205 = call <vilib>:"Application Directory.vi"() -> ("Application Directory"=w167:path)
              n206 = Build Path(base path=w173, name or relative path=w169) -> (appended path=w175:path)
              n207 = Number To Decimal String(number=w164) -> (decimal integer string=w168:string)  [unwired: 1 in]
              n208 = Concatenate Strings(w195, "," ("字符串"), w177, "," ("字符串"), w170) -> (→"单帧部分":string)
              n209 = Build Path(base path=w167, name or relative path="叠加实际" ("名称或相对路径")) -> (appended path=w165:path)
              n210 = Write to Text File(file (use dialog)=w158, text=w157) -> ()  [unwired: 2 in, 3 out]
              n211 = Concatenate Strings(w187, "," ("字符串"), w157, "," ("字符串"), w156) -> (→"叠加部分":string)
              n212 = Write to Text File(file (use dialog)=w175, text=w170) -> ()  [unwired: 2 in, 3 out]
              n213 = Build Path(base path=w165, name or relative path=w168) -> (appended path=w155:path)
              n214 = Write to Text File(file (use dialog)=w155, text=w156) -> ()  [unwired: 2 in, 3 out]
            }
            n215 = case shown="真" w92 {
              frame False {
              }
              frame True {
                n216 = property on="重新选择" class="Bool (严格)"("DisabledEnum"=T2."Enabled" ("禁用")) -> ()  [unwired: 2 in, 2 out]
              }
            }
            n217 = call "IMAQ Dispose"("Image"=w101, "error in (no error)"=w103) -> ("error out"=w102:errorcluster)  [unwired: 1 in, 3 out]
            n218 = call "IMAQ Dispose"("Image"=w110, "error in (no error)"=w102) -> ("error out"=w117:errorcluster)  [unwired: 1 in, 3 out]
            n219 = call "IMAQ Dispose"("Image"=w118, "error in (no error)"=w117) -> ("error out"=w116:errorcluster)  [unwired: 1 in, 3 out]
            n220 = call "IMAQ AVI2 Close"("error in (no error)"=w116, "AVI Refnum"=w146) -> ("error out"=w142:errorcluster)  [unwired: 9 out]
            n221 = call "IMAQ Dispose"("Image"=w141, "error in (no error)"=w142) -> ("error out"=w115:errorcluster)  [unwired: 1 in, 3 out]
            n222 = call "IMAQ Dispose"("error in (no error)"=w115) -> ("error out"=w114:errorcluster)  [unwired: 2 in, 3 out]
            n223 = call <vilib>:"Simple Error Handler.vi"("type of dialog (OK msg:1)"=w94, "error in (no error)"=w114) -> ("error?"=w93:bool)  [unwired: 3 in, 4 out]
            n224 = case shown="真" w93 {
              frame False {
              }
              frame True {
                n225 = property on="重新选择" class="Bool (严格)"("DisabledEnum"=T2."Enabled" ("禁用")) -> ()  [unwired: 2 in, 2 out]
              }
            }
            n226 = local write "重新选择"(FALSE ("重新选择")) -> ()
          }
        }
      }
    }
  }
  "是否进行像素标定" <- FALSE ("是否进行像素标定")
